vi "StepperMotorAngleControl.vi"(7 "stop":bool, 8 "error in":errorcluster, 10 "microstep":dbl=4.0 format="%#_13g", 11 "angle":dbl format="%#_13g") -> (0 "error out":errorcluster)   [LabVIEW 2019]
uses:
  <vilib>/Platform/TimedLoop/XDataNode/timing_clust.ctl
  <vilib>/Platform/TimedLoop/XDataNode/nitl_modes.ctl
  <vilib>/Platform/TimedLoop/XDataNode/wakeup.ctl
  <vilib>/Platform/TimedLoop/XDataNode/XDataNode.xnode
  KNRm_ReMi_OS6_436Motor.lvlibp
  <vilib>/Platform/TimedLoop/XDataNode/XDNodeRunTimeDep.lvlib
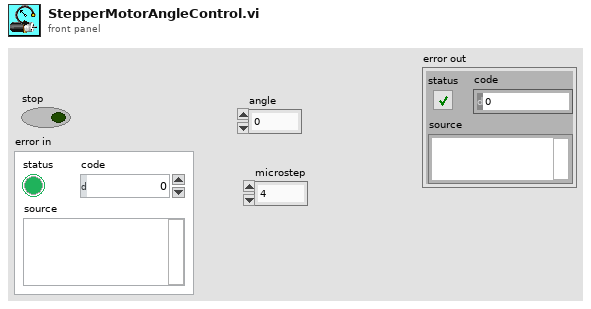
[diagram p1: front panel]
types:
  T1 = typedef "XDNodeRunTimeDep.lvlib/timing_clust.ctl" = cluster{"Expected End [f-1]":u64, "Actual End [f-1]":u64, "Finished Late? [f-1]":bool, "Expected End [i-1]":u64, "Actual End [i-1]":u64, "Finished Late? [i-1]":bool, "Expected Start [i]":u64, "Actual Start [i]":u64, "Expected Start [f]":u64, "Actual Start [f]":u64, "Source Name":string, "Structure Name":string, "Period":i64, "Deadline":i64, "Offset":i64, "Start":i64, "Priority":i32, "Timeout":i32, "Mode":T2, "Wakeup Reason":T3, "Error":errorcluster, "Source Type":string, "Secondary Source Type":string, "Global End Time":u64, "Global Start Time":u64, "Frame Duration":u64, "Iteration Duration":u64, "Assigned CPU":i32, "I/O Scan Engine Mode":u32}
  T2 = typedef "XDNodeRunTimeDep.lvlib/nitl_modes.ctl" = enum32{"No Change", "Process missed periods, maintain original phase", "Discard missed periods, maintain original phase", "Process missed periods, ignore original phase", "Discard missed periods, ignore original phase"}
  T3 = typedef "XDNodeRunTimeDep.lvlib/wakeup.ctl" = enum32{"Normal", "Aborted", "Asynchronous wakeup", "Timing source error", "Timed loop error", "Timeout"}
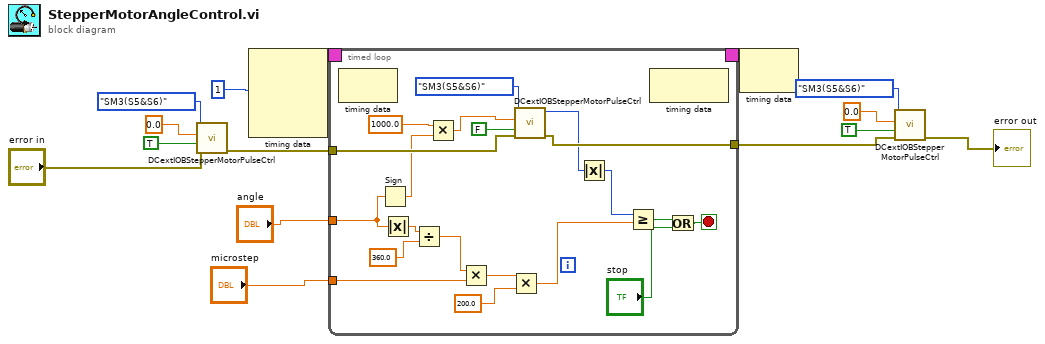
[diagram p0: block diagram]
diagram:
  n1 = call "DCextIOBStepperMotorPulseCtrl.vi"("error in"="error in", "ResetCounter"=TRUE, "PulseRate&Dir P/S"=0.0, "Port"=enum16{"SM1(S1&S2)", "SM2(S3&S4)", "SM3(S5&S6)"}."SM3(S5&S6)") -> ("error out"=w9:errorcluster)  [unwired: 6 in, 1 out]
  n2 = node-c288(i64 1 ("Period")) -> (w12:T1)  [unwired: 3 in]
  n3 = timed-loop {
    timing: w12 -> [_]
    timing-out: [_] -> w11
    tunnel: w9 -> [w33]
    tunnel: [w32] -> w5
    tunnel: "angle" -> [w21]
    tunnel: "microstep" -> [w17]
    stop <- w24 stop-if-true
    n4 = node-c288() -> ()  [unwired: 1 in, 1 out]
    n5 = Sign(1:w21) -> (0:w29:dbl)
    n6 = Absolute Value(x=w21) -> (abs(x)=w20:dbl)
    n7 = Divide(x=w20, y=360.0) -> (x/y=w18:dbl)
    n8 = Multiply(x=1000.0 ("PulseRate&Dir P/S"), y=w29) -> (x*y=w27:dbl)
    n9 = Multiply(x=w18, y=w17) -> (x*y=w31:dbl)
    n10 = Multiply(x=w31, y=200.0) -> (x*y=w23:dbl)
    n11 = call "DCextIOBStepperMotorPulseCtrl.vi"("error in"=w33, "ResetCounter"=FALSE, "PulseRate&Dir P/S"=w27, "Port"=enum16{"SM1(S1&S2)", "SM2(S3&S4)", "SM3(S5&S6)"}."SM3(S5&S6)") -> ("error out"=w32:errorcluster, "PulseCounter+/-"=w26:i32)  [unwired: 6 in]
    n12 = Absolute Value(x=w26) -> (abs(x)=w25:i32)
    n13 = Greater Or Equal?(x=w25, y=w23) -> (x >= y?=w22:bool)
    n14 = node-c288() -> ()  [unwired: 1 in, 1 out]
    n15 = Or(x=w22, y="stop") -> (x .or. y?=w24:bool)
  }
  n16 = node-c288(w11) -> ()  [unwired: 1 out]
  n17 = call "DCextIOBStepperMotorPulseCtrl.vi"("error in"=w5, "ResetCounter"=TRUE, "PulseRate&Dir P/S"=0.0, "Port"=enum16{"SM1(S1&S2)", "SM2(S3&S4)", "SM3(S5&S6)"}."SM3(S5&S6)") -> ("error out"=→"error out":errorcluster)  [unwired: 6 in, 1 out]
